vi "armCamera.vi"(0 "Camera in":refnum<class "Camera.lvclass">, 11 "error in (no error)":errorcluster) -> (4 "Camera out":refnum<class "Camera.lvclass">, 15 "error out":errorcluster)   [LabVIEW 2019, in "Camera.lvclass"]
doc: "Calculates the current color mode.\nThis means, according to the current roi and the color pattern of the camera, determin whih color is on the top left pixel of the image.\nThis is needed for correct debayering"
uses:
  Camera.lvclass
  Camera.lvclass/Camera.ctl
  pco.sdk/GeneralCameraControl/GeneralCameraControl.lvlib
  pco.sdk/GeneralCameraStatus/GeneralCameraStatus.lvlib
  pco.sdk/CameraDescription/CameraDescription.lvlib
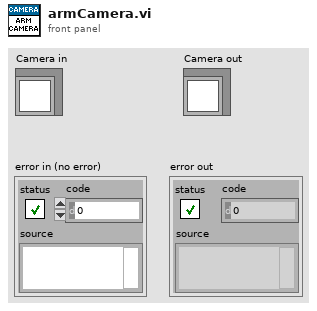
[diagram p1: front panel]
types:
  T1 = cluster{"wSensorTypeDESC":u16, "wSensorSubTypeDESC":u16, "wMaxHorzResStdDESC":u16, "wMaxVertResStdDESC":u16, "wMaxHorzResExtDESC":u16, "wMaxVertResExtDESC":u16, "wDynResDESC":u16, "wMaxBinHorzDESC":u16, "wBinHorzSteppingDESC":u16, "wMaxBinVertDESC":u16, "wBinVertSteppingDESC":u16, "wRoiHorStepsDESC":u16, "wRoiVertStepsDESC":u16, "wNumADCsDESC":u16, "wMinSizeHorzDESC":u16, "dwPixelRateDESC":u32[], "wConvFactDESC":u16[], "sCoolingSetpoints":i16[], "wSoftRoiHorStepsDESC":u16, "wSoftRoiVertStepsDESC":u16, "wIRDESC":u16, "wMinSizeVertDESC":u16, "dwMinDelayDESC":u32, "dwMaxDelayDESC":u32, "dwMinDelayStepDESC":u32, "dwMinExposureDESC":u32, "dwMaxExposureDESC":u32, "dwMinExposureStepDESC":u32, "dwMinDelayIRDESC":u32, "dwMaxDelayIRDESC":u32, "dwMinExposureIRDESC":u32, "dwMaxExposureIRDESC":u32, "wTimeTableDESC":u16, "wDoubleImageDESC":u16, "sMinCoolSetDESC":i16, "sMaxCoolSetDESC":i16, "sDefaultCoolSetDESC":i16, "wPowerDownModeDESC":u16, "wOffsetRegulationDESC":u16, "wColorPatternDESC":u16, "wPatternTypeDESC":u16, "wNumCoolingSetpoints":u16, "dwGeneralCapsDESC1":u32, "dwGeneralCapsDESC2":u32, "dwExtSyncFrequency":u32[], "dwGeneralCapsDESC3":u32, "dwGeneralCapsDESC4":u32}
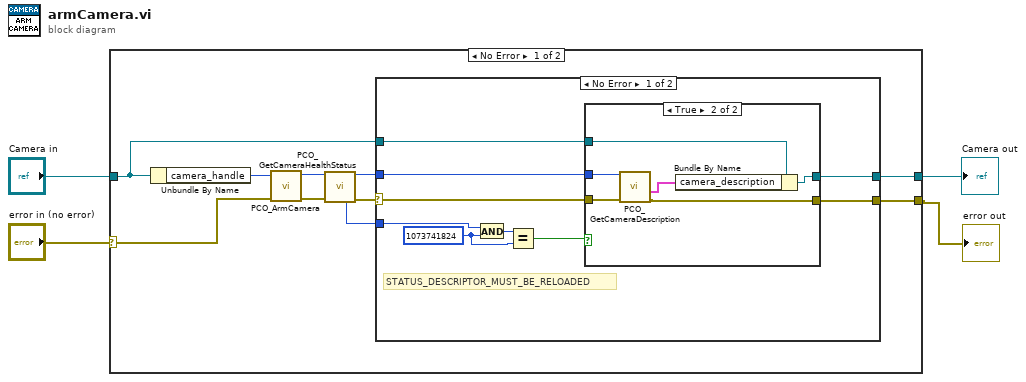
[diagram p0: block diagram]
diagram:
  n1 = case shown="No Error" "error in (no error)" {
    selector: "error in (no error)" -> [w13 w34]
    tunnel: [w5 w35] -> w3
    tunnel: "Camera in" -> [w7 w35]
    tunnel: [w6 w34] -> w1
    frame No Error {
      n2 = Unbundle By Name(w7) -> ("camera_handle"=w14:u64)
      n3 = call "PCO_ArmCamera.vi"("error in (no error)"=w13, "ph"=w14) -> ("error out"=w11:errorcluster, "ph out"=w12:u64)  [unwired: 7 in, 1 out]
      n4 = call "PCO_GetCameraHealthStatus.vi"("ph"=w12, "error in (no error)"=w11) -> ("ph out"=w8:u64, "dwStatus"=w9:u32, "error out"=w10:errorcluster)  [unwired: 8 in, 3 out]
      n5 = case shown="No Error" w10 {
        selector: w10 -> [w19 w32]
        tunnel: w9 -> [w23 _]
        tunnel: w8 -> [w18 _]
        tunnel: w7 -> [w17 w33]
        tunnel: [w16 w32] -> w6
        tunnel: [w15 w33] -> w5
        frame No Error {
          w21 = u32 1073741824 ("y")
          # "STATUS_DESCRIPTOR_MUST_BE_RELOADED"
          n6 = And(x=w23, y=w21) -> (x .and. y?=w22:u32)
          n7 = Equal?(x=w22, y=w21) -> (x = y?=w20:bool)
          n8 = case shown="True" w20 {
            tunnel: w19 -> [w24 w31]
            tunnel: w18 -> [_ w30]
            tunnel: w17 -> [w25 w29]
            tunnel: [w24 w27] -> w16
            tunnel: [w25 w26] -> w15
            frame False {
            }
            frame True {
              n9 = call "PCO_GetCameraDescription.vi"("error in (no error)"=w31, "ph"=w30) -> ("error out"=w27:errorcluster, "strDescription"=w28:T1)  [unwired: 6 in, 2 out]
              n10 = Bundle By Name(cluster=w29, "camera_description"=w28) -> (w26:refnum<class "Camera.lvclass">)
            }
          }
        }
        frame Error {
        }
      }
    }
    frame Error {
    }
  }
  "error out" <- w1
  "Camera out" <- w3
